vi "Controller - NStream Read.vi"(8 "error in (no error)":errorcluster, 11 "View Model":T1) -> (0 "error out":errorcluster, 1 "Total Elements":u64, 2 "Available Elmnts":i32, 3 "View Model":T1)   [LabVIEW 2017]
doc: "This SubVI provides data processing from NW Stream\ninto 2D RT data array in DVR"
uses:
  View Model/Controls/View Model.ctl
  View Model/Controls/Shared Model.ctl
  Error Handler/Controls/Error Model.ctl
  Error Handler/Controls/Error Event.ctl
  Error Handler/Controls/Error Type.ctl
  Controls/Controller Model.ctl
  Controls/Controller Event.ctl
  Controls/Controller Command.ctl
  Controls/Controller Overhead.ctl
  Real-Time/RT Status.ctl
  Real-Time/RT Loop Status.ctl
  Controls/Controller NStream.ctl
  Controls/Controller Timer Data.ctl
  Controls/Controller DAQ Data.ctl
  TDMS Logger/Controls/TDMS Model.ctl
  TDMS Logger/Controls/TDMS Event.ctl
  TDMS Logger/Controls/TDMS Command.ctl
  TDMS Logger/Controls/TDMS Overhead.ctl
  TDMS Logger/Controls/TDMS ChanProperties.ctl
  TDMS Logger/Controls/TDMS DAQ Data.ctl
  <resource>/objmgr/ni.dex.rc
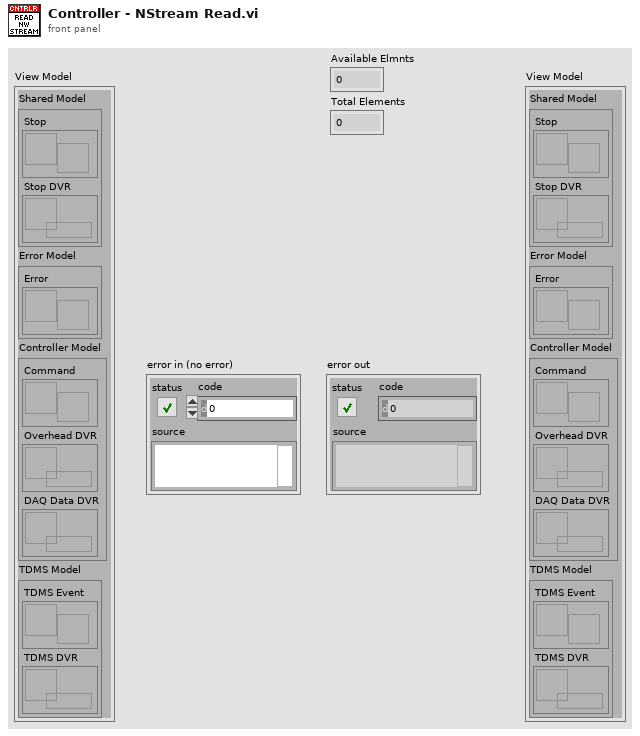
[diagram p1: front panel]
types:
  T1 = typedef "View Model.ctl" = cluster{"Shared Model":T2, "Error Model":T3, "Controller Model":T4, "TDMS Model":T5}
  T2 = typedef "Shared Model.ctl" = cluster{"Stop":refnum<user-event>, "Stop DVR":refnum<data-value>}
  T3 = typedef "Error Model.ctl" = cluster{"Error":refnum<user-event>}
  T4 = typedef "Controller Model.ctl" = cluster{"Command":refnum<user-event>, "Overhead DVR":refnum<data-value>, "DAQ Data DVR":refnum<data-value>}
  T5 = typedef "TDMS Model.ctl" = cluster{"TDMS Event":refnum<user-event>, "TDMS DVR":refnum<data-value>}
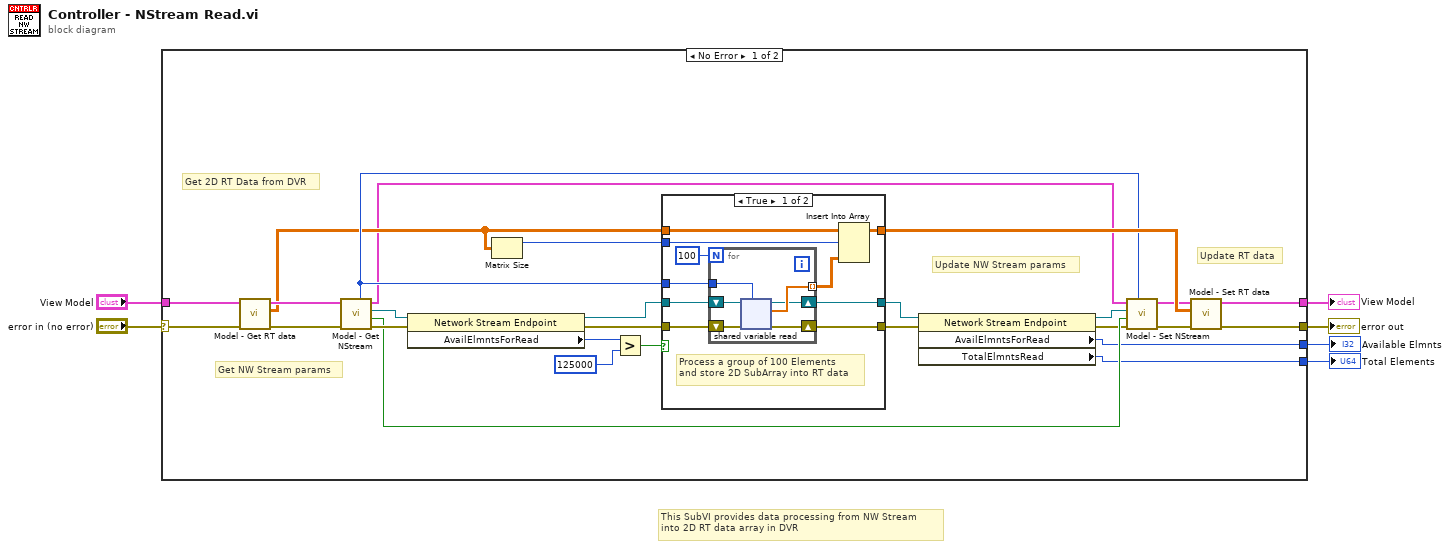
[diagram p0: block diagram]
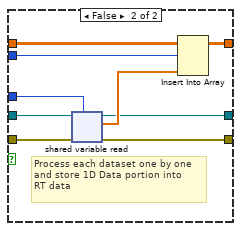
[diagram p2: hidden frame]
diagram:
  # "This SubVI provides data processing from NW Stream\ninto 2D RT data array in DVR"
  n1 = case shown="No Error" "error in (no error)" {
    selector: "error in (no error)" -> [w16 w59]
    tunnel: [w10 w59] -> w5
    tunnel: "View Model" -> [w15 w60]
    tunnel: [w11 w60] -> w3
    tunnel: [w9 _] -> w2
    tunnel: [w8 _] -> w1
    frame No Error {
      # "Update RT data"
      # "Update NW Stream params"
      # "Get NW Stream params"
      # "Get 2D RT Data from DVR"
      n2 = call "Model - Get RT data.vi"("error in (no error)"=w16, "View Model"=w15) -> ("error out"=w18:errorcluster, "RT data"=w14:dbl[][], "View Model"=w17:T1)  [unwired: 7 in]
      n3 = call "Model - Get NStream.vi"("error in (no error)"=w18, "View Model"=w17) -> ("error out"=w32:errorcluster, "exist?"=w26:bool, "Endpoint"=w33:refnum<k21>, "View Model"=w7:T1, "RTDataElmnts"=w19:i32)  [unwired: 4 in, 1 out]
      n4 = property class="Network Stream Endpoint"(reference=w33, error in=w32) -> (reference out=w30:refnum<k21>, error out=w31:errorcluster, "AvailElmntsForRead"=w24:i32)
      n5 = Matrix Size(0:w14) -> (1:w27:i32)  [unwired: 1 out]
      n6 = Greater?(x=w24, y=125000) -> (0:w28:bool)
      n7 = case shown="True" w28 {
        tunnel: w19 -> [w43 w58]
        tunnel: [w42 w57] -> w22
        tunnel: w31 -> [w41 w56]
        tunnel: w30 -> [w40 w55]
        tunnel: w27 -> [w39 w54]
        tunnel: [w37 w52] -> w25
        tunnel: w14 -> [w36 w51]
        tunnel: [w35 w50] -> w23
        frame True {
          # "Process a group of 100 Elements\nand store 2D SubArray into RT data"
          n8 = for {
            N: 100 -> [_]
            tunnel: [w47] -> w38 mode=indexing
            tunnel: w43 -> [w46]
            shift-right: [w44] -> w35
            shift-left: w40 -> [w48]
            shift-right: [w45] -> w42
            shift-left: w41 -> [w49]
            n9 = shared-variable-read(w48, w49, w46) -> (w44:refnum<k21>, w45:errorcluster, w47:dbl[])  [unwired: 1 in, 1 out]
          }
          n10 = Insert Into Array(array=w36, index (row)=w39, new element=w38) -> (w37:dbl[][])  [unwired: 1 in]
        }
        frame False {
          # "Process each dataset one by one\nand store 1D Data portion into\nRT data"
          n11 = shared-variable-read(w55, w56, w58) -> (w50:refnum<k21>, w57:errorcluster, w53:dbl[])  [unwired: 1 in, 1 out]
          n12 = Insert Into Array(array=w51, index (row)=w54, new element=w53) -> (w52:dbl[][])  [unwired: 1 in]
        }
      }
      n13 = property class="Network Stream Endpoint"(reference=w23, error in=w22) -> (reference out=w21:refnum<k21>, error out=w20:errorcluster, "AvailElmntsForRead"=w9:i32, "TotalElmntsRead"=w8:u64)
      n14 = call "Model - Set NStream.vi"("RTDataElmnts"=w19, "error in (no error)"=w20, "exist?"=w26, "Endpoint"=w21, "View Model"=w7) -> ("error out"=w12:errorcluster, "View Model"=w13:T1)  [unwired: 5 in]
      n15 = call "Model - Set RT data.vi"("error in (no error)"=w12, "RT data"=w25, "View Model"=w13) -> ("error out"=w10:errorcluster, "View Model"=w11:T1)  [unwired: 7 in]
    }
    frame Error {
    }
  }
  "View Model" <- w3
  "error out" <- w5
  "Available Elmnts" <- w2
  "Total Elements" <- w1
